vi "Get Font.vi"(8 "error in":errorcluster, 11 "View in":refnum<class "Cell View.lvclass">) -> (0 "error out":errorcluster, 2 "Font.lvclass":refnum<class "Font.lvclass">, 3 "View out":refnum<class "Cell View.lvclass">)   [LabVIEW 2023, in "SourceGrid.lvlib" / "Cell View.lvclass"]
uses:
  Cell View.lvclass
  Font/Font.lvclass
  Cell View.lvclass/Cell View.ctl
  D:/git/Sourcegrid-LabVIEW/dll/SourceGrid.dll
  dll/SourceGrid.dll
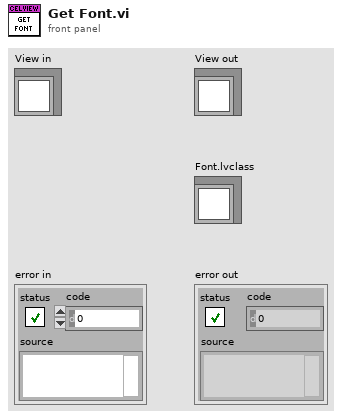
[diagram p1: front panel]
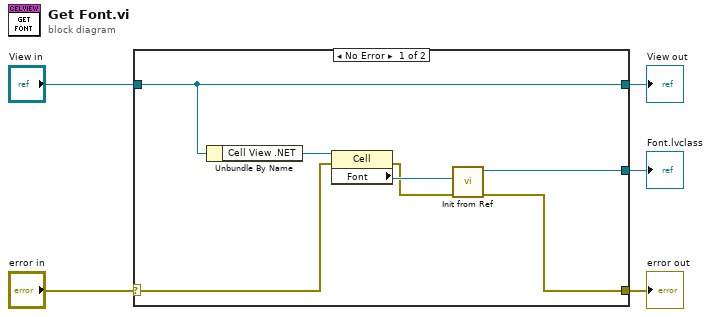
[diagram p0: block diagram]
diagram:
  n1 = case shown="No Error" "error in" {
    selector: "error in" -> [w12 w13]
    tunnel: [w8 w13] -> w4
    tunnel: [w11 w14] -> w2
    tunnel: "View in" -> [w11 w14]
    tunnel: [w7 _] -> w1
    frame No Error {
      n2 = Unbundle By Name(w11) -> ("Cell View .NET"=w6:refnum<k24>)
      n3 = property class="Cell"(reference=w6, error in=w12) -> (error out=w9:errorcluster, "Font"=w10:refnum<k24>)  [unwired: 1 out]
      n4 = call "Init from Ref.vi"("error in"=w9, "Font"=w10) -> ("error out"=w8:errorcluster, "Font out"=w7:refnum<class "Font.lvclass">)  [unwired: 8 in]
    }
    frame Error {
    }
  }
  "error out" <- w4
  "View out" <- w2
  "Font.lvclass" <- w1
